vi "Player Info.vi"(11 "MRM Clones in":refnum<class "MRM Clones.lvclass">) -> (0 "Defeat Speech":string, 1 "Victory Speech":string, 2 "Name":string, 3 "MRM Clones out":refnum<class "MRM Clones.lvclass">)   [LabVIEW 2016, in "MRM Clones.lvclass"]
uses:
  MRM Clones.lvclass
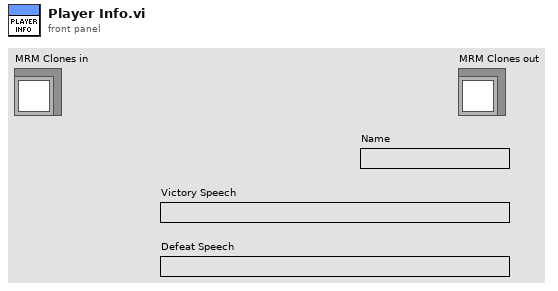
[diagram p1: front panel]
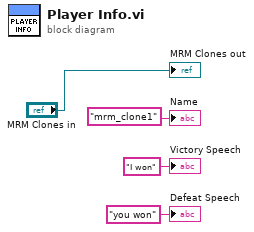
[diagram p0: block diagram]
diagram:
  "MRM Clones out" <- "MRM Clones in"
  "Name" <- "mrm_clone1" ("Name")
  "Victory Speech" <- "I won" ("Victory Speech")
  "Defeat Speech" <- "you won" ("Defeat Speech")
